vi "CMCryoControl.vi"() -> ()   [LabVIEW 2017]
uses:
  Globals/globals.vi
  Commands/ScanInterfaceGlobalData.vi
  Types/ScanInfo.ctl
panel:
  in  "Tab Control":enum32{"Control", "Measurements", "Defenitions"}(tab)
  in  "positionTrack":bool=TRUE
  in  "positionGO":bool
  in  "Position Info":cluster{"X":dbl, "Y":dbl} {"Y" step=0.01; "X" step=0.01}
  in  "StartStream":bool
  in  "Scan Info":T1={"X Center"=0.0, "Y Center"=0.0, "Width"=1.0, "Height"=1.0, "Time [ms]"=1000.0, "As Dwell Time"=FALSE, "Pixels"=1000.0}
  in  "ScanBtn":bool
  in  "Experiment List":i32(listbox)
  in  "Experiment Grps":u16(ring) items=["Sequential", "Time Resolved"]
  in  "StreamRate":dbl=10000.0
  in  "VI Search Path":path=path "C:/Code/CMCryoSysLabView/Experiments"
  out "CurrentReadAmplitude":dbl=50.013
  in  "Notifiers":T2
  out "Working":bool
  in  "IntensitySave":bool
  in  "IntensityLogScale":bool
  out "ScanImage":dbl[][](graph)
  in  "StreamSave":bool
  in  "StreamLogScale":bool
  out "Counter Trace":waveform(dbl)(graph)={"t0"=timestamp(1099.9 s since 1904-01-01), "dt"=0.09999999999990905, "Y"=array[30001 elements]}
  # "Dbl click to open experiment (or select and press open)"
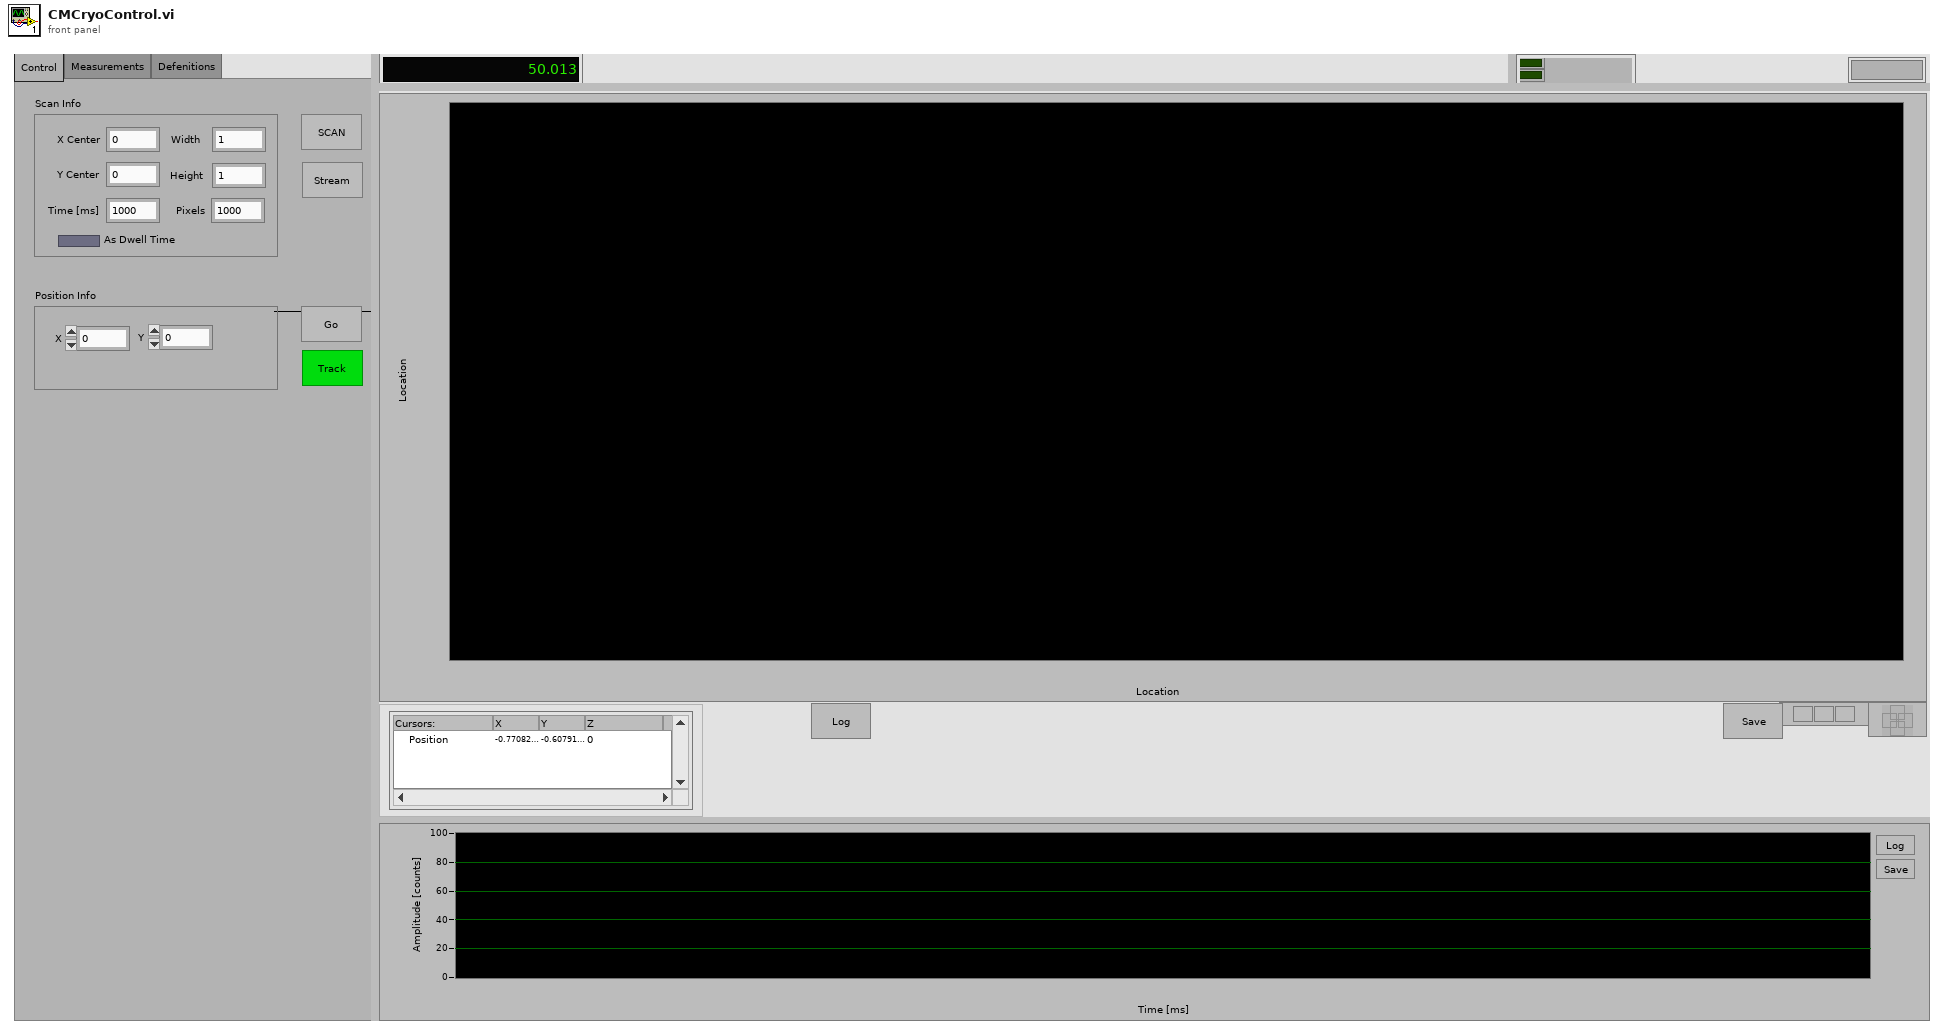
[diagram p1: front panel]
types:
  T1 = typedef "ScanInfo.ctl" = cluster{"X Center":dbl, "Y Center":dbl, "Width":dbl, "Height":dbl, "Time [ms]":dbl, "As Dwell Time":bool, "Pixels":dbl}
  T2 = cluster{"ImageCompleted":bool, "ImageUpdated":bool}
  T3 = typedef "ExperimentGrp.ctl" = cluster{"Path":path, "Experiments":path[], "Name":string, "Experiment Names":string[]}
  T4 = typedef "NotificationsInfo.ctl" = cluster{"ImageComplete":bool}
  T5 = typedef "StreamInfo.ctl" = cluster{"Waveform":waveform(dbl), "isNew":bool, "MeanV":dbl}
  T6 = typedef "ImageInfo.ctl" = cluster{"IsNew":bool, "Data":dbl[][], "XOffset":dbl, "YOffset":dbl, "dy":dbl, "dx":dbl, "xmin":dbl, "xmax":dbl, "ymin":dbl, "ymax":dbl, "width":dbl, "height":dbl, "whRatio":dbl}
  T7 = typedef "LVPoint32TypeDef.ctl" = cluster{"Horizontal":i32, "Vertical":i32}
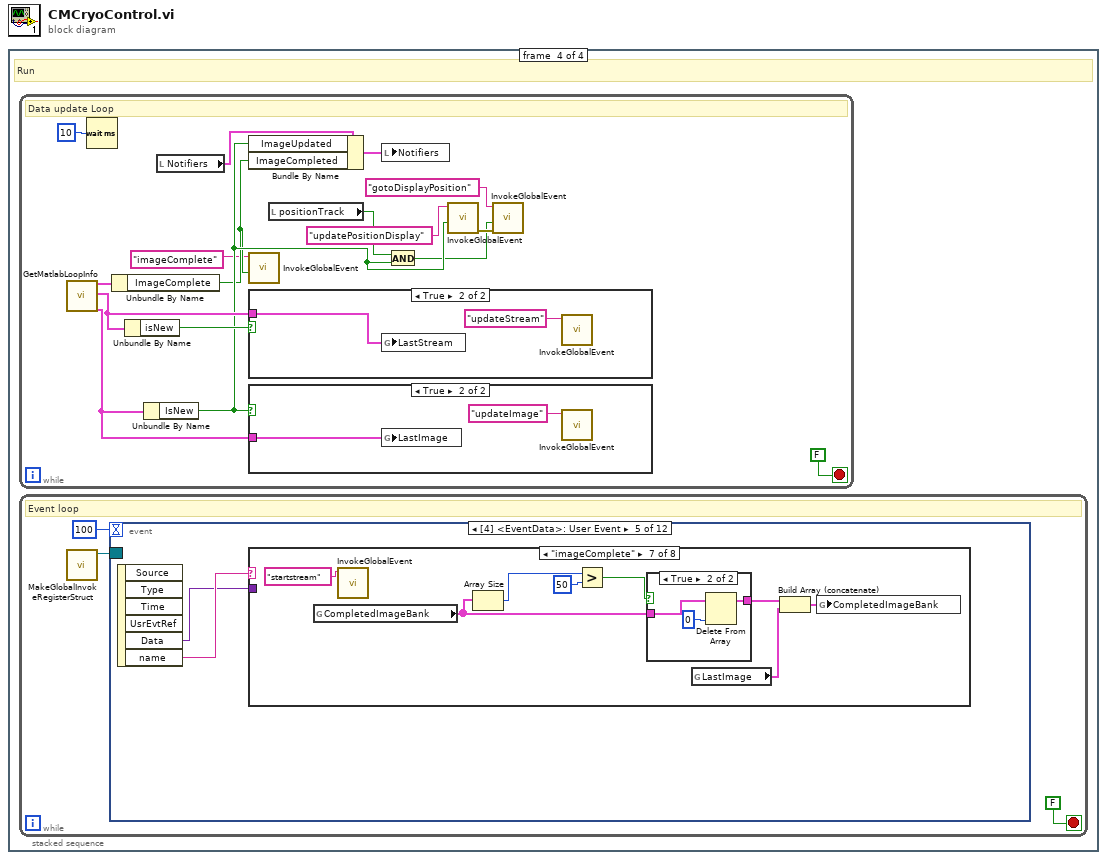
[diagram p0: block diagram]
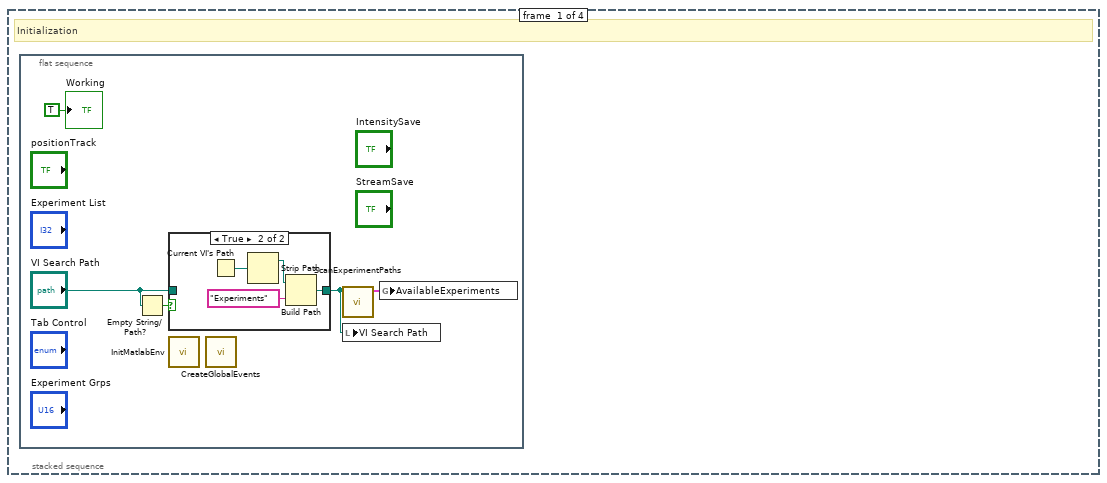
[diagram p2: hidden frame]
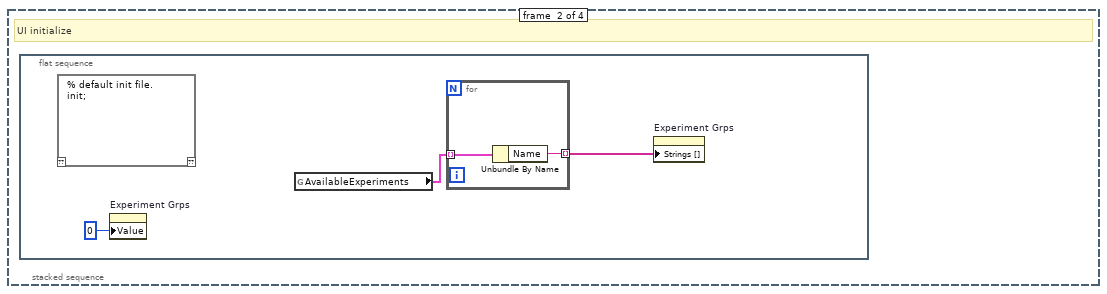
[diagram p4: hidden frame]
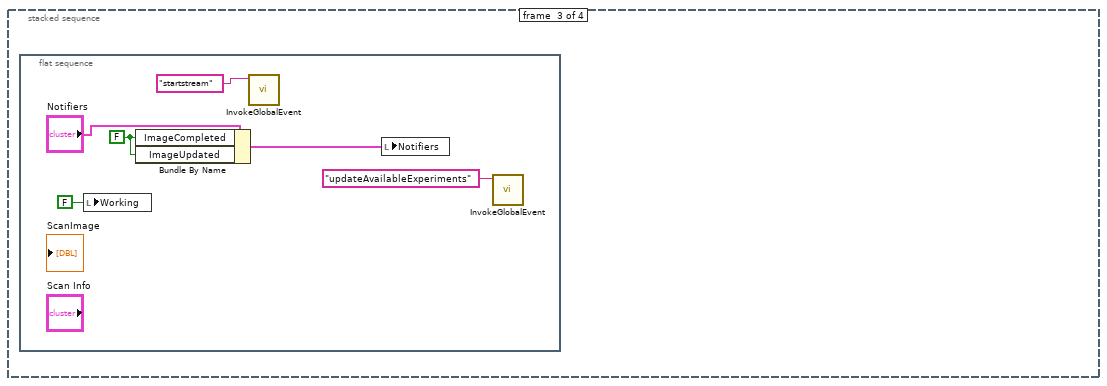
[diagram p5: hidden frame]
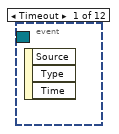
[diagram p8: hidden frame]
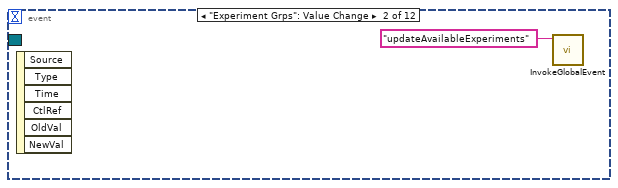
[diagram p9: hidden frame]
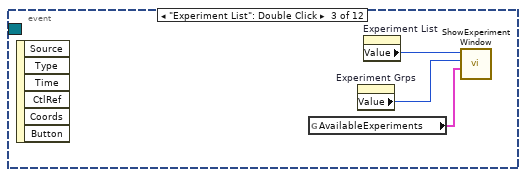
[diagram p10: hidden frame]
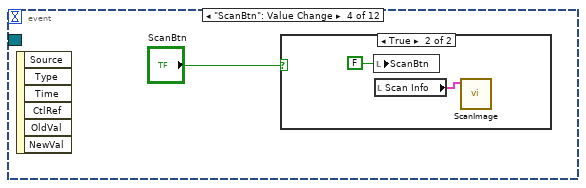
[diagram p11: hidden frame]
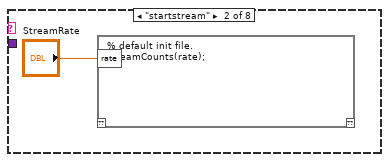
[diagram p14: hidden frame]
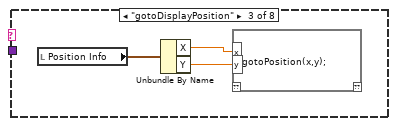
[diagram p15: hidden frame]
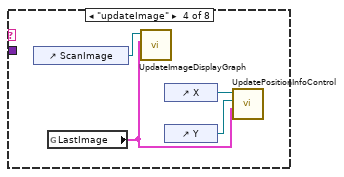
[diagram p16: hidden frame]
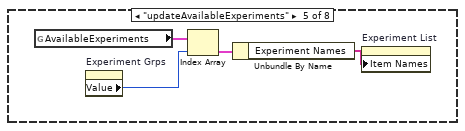
[diagram p17: hidden frame]
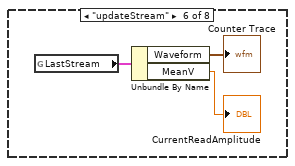
[diagram p18: hidden frame]
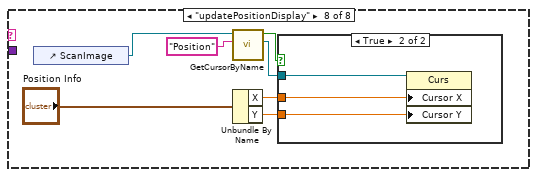
[diagram p20: hidden frame]
diagram:
  n1 = stacked-sequence {
    frame #0 {
      # "Initialization"
      n2 = flat-sequence {
        frame #0 {
          n3 = Empty String/Path?(string/path="VI Search Path") -> (empty?=w4:bool)
          n4 = case shown="True" w4 {
            tunnel: [w6 w8] -> w3
            tunnel: "VI Search Path" -> [w6 _]
            frame False {
            }
            frame True {
              n5 = Current VI's Path() -> (path=w7:path)
              n6 = Strip Path(path=w7) -> (stripped path=w10:path)  [unwired: 1 out]
              n7 = Build Path(base path=w10, name or relative path="Experiments") -> (appended path=w8:path)
            }
          }
          n8 = call "InitMatlabEnv.vi"() -> ()  [unwired: 12 in]
          n9 = call "CreateGlobalEvents.vi"() -> ()  [unwired: 12 in]
          n10 = call "ScanExperimentPaths.vi"("Scan path"=w3) -> ("AvailableExperiments"=w2:T3[])  [unwired: 10 in]
          n11 = local write "VI Search Path"(w3) -> ()
          n12 = global write "globals.vi" "AvailableExperiments"(w2) -> ()
          "Working" <- TRUE ("Status")
        }
      }
    }
    frame #1 {
      # "UI initialize"
      n13 = flat-sequence {
        frame #0 {
          n14 = script code="% default init file.\ninit;"() -> ()  [unwired: 1 in, 1 out]
          n15 = property on="Experiment Grps" class="Ring (strict)"("Value"=0 ("index")) -> ()  [unwired: 2 in, 2 out]
          n16 = global read "globals.vi" "AvailableExperiments"() -> (w13:T3[])
          n17 = for {
            tunnel: w13 -> [w15] mode=indexing
            tunnel: [w14] -> w12 mode=indexing
            n18 = Unbundle By Name(w15) -> ("Name"=w14:string)
          }
          n19 = property on="Experiment Grps" class="Ring (strict)"("Strings []"=w12) -> ()  [unwired: 2 in, 2 out]
        }
      }
    }
    frame #2 {
      n20 = flat-sequence {
        frame #0 {
          w19 = FALSE ("ImageCompleted")
          n21 = local write "Working"(FALSE ("Working")) -> ()
          n22 = Bundle By Name(cluster="Notifiers", "ImageCompleted"=w19, "ImageUpdated"=w19) -> (w20:T2)
          n23 = call "InvokeGlobalEvent.vi"("name"="startstream" ("event data")) -> ()  [unwired: 10 in, 1 out]
          n24 = local write "Notifiers"(w20) -> ()
          n25 = call "InvokeGlobalEvent.vi"("name"="updateAvailableExperiments" ("event data")) -> ()  [unwired: 10 in, 1 out]
        }
      }
    }
    frame #3 {
      # "Run"
      n26 = while {
        stop <- FALSE stop-if-true
        # "Data update Loop"
        n27 = call "GetMatlabLoopInfo.vi"() -> ("Notifications"=w33:T4, "StreamInfo"=w30:T5, "ImageInfo"=w29:T6)  [unwired: 17 in]
        n28 = Wait (ms)(milliseconds to wait=u32 10) -> ()  [unwired: 1 out]
        n29 = Unbundle By Name(w33) -> ("ImageComplete"=w23:bool)
        n30 = Unbundle By Name(w30) -> ("isNew"=w28:bool)
        n31 = Unbundle By Name(w29) -> ("IsNew"=w27:bool)
        n32 = local read "Notifiers"() -> (w35:T2)
        n33 = Bundle By Name(cluster=w35, "ImageUpdated"=w27, "ImageCompleted"=w23) -> (w34:T2)
        n34 = call "InvokeGlobalEvent.vi"("Invoke?"=w23, "name"="imageComplete" ("event data")) -> ()  [unwired: 9 in, 1 out]
        n35 = case shown="True" w28 {
          tunnel: w30 -> [_ w41]
          frame False {
          }
          frame True {
            n36 = global write "ScanInterfaceGlobalData.vi" "LastStream"(w41) -> ()
            n37 = call "InvokeGlobalEvent.vi"("name"="updateStream" ("event data")) -> ()  [unwired: 10 in, 1 out]
          }
        }
        n38 = case shown="True" w27 {
          tunnel: w29 -> [_ w39]
          frame False {
          }
          frame True {
            n39 = global write "ScanInterfaceGlobalData.vi" "LastImage"(w39) -> ()
            n40 = call "InvokeGlobalEvent.vi"("name"="updateImage" ("event data")) -> ()  [unwired: 10 in, 1 out]
          }
        }
        n41 = local read "positionTrack"() -> (w32:bool)
        n42 = local write "Notifiers"(w34) -> ()
        n43 = And(x=w32, y=w27) -> (x .and. y?=w26:bool)
        n44 = call "InvokeGlobalEvent.vi"("Invoke?"=w27, "name"="updatePositionDisplay" ("event data")) -> ("error out"=w31:errorcluster)  [unwired: 9 in]
        n45 = call "InvokeGlobalEvent.vi"("error in (no error)"=w31, "Invoke?"=w26, "name"="gotoDisplayPosition" ("event data")) -> ()  [unwired: 8 in, 1 out]
      }
      n46 = while {
        stop <- FALSE stop-if-true
        # "Event loop"
        n47 = call "MakeGlobalInvokeRegisterStruct.vi"() -> ("Event Registration Refnum out"=w42:refnum<event-registration>)  [unwired: 11 in]
        n48 = event shown="[4] <EventData>: User Event" {
          selector: w42 -> [_ _ _ _ _ _ _ _ _ _ _ _]
          dyn-events: _ -> [_ _ _ _ _ _ _ _ _ _ _ _]
          timeout: 100 -> [_ _ _ _ _ _ _ _ _ _ _ _]
          event Timeout {
            n49 = event-data() -> ()  [unwired: 1 in, 3 out]
          }
          event "Experiment Grps": Value Change {
            n50 = event-data() -> ()  [unwired: 1 in, 6 out]
            n51 = call "InvokeGlobalEvent.vi"("name"="updateAvailableExperiments" ("event data")) -> ()  [unwired: 10 in, 1 out]
          }
          event "Experiment List": Double Click {
            n52 = event-data() -> ()  [unwired: 1 in, 6 out]
            n53 = global read "globals.vi" "AvailableExperiments"() -> (w48:T3[])
            n54 = property on="Experiment Grps" class="Ring (strict)"() -> ("Value"=w46:u16)  [unwired: 2 in, 2 out]
            n55 = property on="Experiment List" class="LstBox (strict)"() -> ("Value"=w47:i32)  [unwired: 2 in, 2 out]
            n56 = call "ShowExperimentWindow.vi"("AvailableExperiments"=w48, "Value"=w46, "Value 2"=w47) -> ()  [unwired: 9 in]
          }
          event "ScanBtn": Value Change {
            n57 = event-data() -> ()  [unwired: 1 in, 6 out]
            n58 = case shown="True" "ScanBtn" {
              frame False {
              }
              frame True {
                n59 = local write "ScanBtn"(FALSE ("ScanBtn")) -> ()
                n60 = local read "Scan Info"() -> (w50:T1)
                n61 = call "ScanImage.vi"("Scan Info"=w50) -> ()  [unwired: 11 in]
              }
            }
          }
          event User Event {
            n62 = event-data() -> ("Data"=w52:variant, "name"=w53:string)  [unwired: 1 in, 4 out]
            n63 = case shown="\"imageComplete\"" w53 {
              tunnel: w52 -> [_ _ _ _ _ _ _ _]
              frame "False", Default {
              }
              frame "startstream" {
                n64 = script code="% default init file.\nstreamCounts(rate);"("rate"="StreamRate") -> ()  [unwired: 1 in, 1 out]
              }
              frame "gotoDisplayPosition" {
                n65 = local read "Position Info"() -> (w57:cluster{"X":dbl, "Y":dbl})
                n66 = Unbundle By Name(w57) -> ("X"=w56:dbl, "Y"=w55:dbl)
                n67 = script code="gotoPosition(x,y);"("x"=w56, "y"=w55) -> ()  [unwired: 1 in, 1 out]
              }
              frame "updateImage" {
                n68 = control-ref of="ScanImage"() -> (w59:refnum<vi>)
                n69 = global read "ScanInterfaceGlobalData.vi" "LastImage"() -> (w58:T6)
                n70 = call "UpdateImageDisplayGraph.vi"("ImageInfo"=w58, "IntensityGraph in"=w59) -> ()  [unwired: 10 in]
                n71 = control-ref of="X"() -> (w60:refnum<vi>)
                n72 = control-ref of="Y"() -> (w61:refnum<vi>)
                n73 = call "UpdatePositionInfoControl.vi"("ImageInfo"=w58, "Y"=w61, "Digital in"=w60) -> ()  [unwired: 9 in]
              }
              frame "updateAvailableExperiments" {
                n74 = global read "globals.vi" "AvailableExperiments"() -> (w63:T3[])
                n75 = property on="Experiment Grps" class="Ring (strict)"() -> ("Value"=w62:u16)  [unwired: 2 in, 2 out]
                n76 = Index Array(array=w63, index=w62) -> (element=w64:T3)
                n77 = Unbundle By Name(w64) -> ("Experiment Names"=w65:string[])
                n78 = property on="Experiment List" class="LstBox (strict)"("Item Names"=w65) -> ()  [unwired: 2 in, 2 out]
              }
              frame "updateStream" {
                n79 = global read "ScanInterfaceGlobalData.vi" "LastStream"() -> (w66:T5)
                n80 = Unbundle By Name(w66) -> ("Waveform"=→"Counter Trace":waveform(dbl), "MeanV"=→"CurrentReadAmplitude":dbl)
              }
              frame "imageComplete" {
                n81 = global read "ScanInterfaceGlobalData.vi" "CompletedImageBank"() -> (w71:T6[])
                n82 = call "InvokeGlobalEvent.vi"("name"="startstream" ("event data")) -> ()  [unwired: 10 in, 1 out]
                n83 = Array Size(array=w71) -> (size(s)=w74:i32)
                n84 = Greater?(x=w74, y=50) -> (0:w72:bool)
                n85 = case shown="True" w72 {
                  tunnel: w71 -> [w77 w80]
                  tunnel: [w77 w78] -> w70
                  frame False {
                  }
                  frame True {
                    n86 = Delete From Array(array=w80, index=0) -> (array with subset deleted=w78:T6[])  [unwired: 1 in, 1 out]
                  }
                }
                n87 = global read "ScanInterfaceGlobalData.vi" "LastImage"() -> (w76:T6)
                n88 = Build Array (concatenate)(w70, w76) -> (w75:T6[])
                n89 = global write "ScanInterfaceGlobalData.vi" "CompletedImageBank"(w75) -> ()
              }
              frame "updatePositionDisplay" {
                n90 = control-ref of="ScanImage"() -> (w87:refnum<vi>)
                n91 = call "GetCursorByName.vi"("Name"="Position", "IntensityGraph in"=w87) -> ("CursorRef"=w82:refnum<vi>, "Found?"=w81:bool)  [unwired: 7 in, 1 out]
                n92 = Unbundle By Name("Position Info") -> ("X"=w84:dbl, "Y"=w83:dbl)
                n93 = case shown="True" w81 {
                  tunnel: w84 -> [_ w90]
                  tunnel: w83 -> [_ w89]
                  tunnel: w82 -> [_ w88]
                  frame False {
                  }
                  frame True {
                    n94 = property class="Curs"(reference=w88, "Cursor X"=w90, "Cursor Y"=w89) -> ()  [unwired: 1 in, 2 out]
                  }
                }
              }
            }
          }
          event "Position Info": Value Change {
            n95 = event-data() -> ()  [unwired: 1 in, 6 out]
            n96 = local read "positionTrack"() -> (w92:bool)
            n97 = call "InvokeGlobalEvent.vi"("name"="updatePositionDisplay" ("event data")) -> ("error out"=w93:errorcluster)  [unwired: 10 in]
            n98 = case shown="True" w92 {
              tunnel: w93 -> [_ _]
              frame False {
              }
              frame True {
                n99 = call "InvokeGlobalEvent.vi"("name"="gotoDisplayPosition" ("event data")) -> ()  [unwired: 10 in, 1 out]
              }
            }
          }
          event "ScanImage": Mouse Up {
            n100 = event-data() -> ("Coords"=w103:T7)  [unwired: 1 in, 7 out]
            n101 = invoke on="ScanImage" class="IntGraph (strict)" method="Map Coords To XY"("Coords"=w103) -> ("XY"=w101:cluster{"X":dbl, "Y":dbl})  [unwired: 6 in, 6 out]
            n102 = local read "positionTrack"() -> (w96:bool)
            n103 = Unbundle By Name(w101) -> ("X"=w100:dbl, "Y"=w99:dbl)
            n104 = local read "Position Info"() -> (w102:cluster{"X":dbl, "Y":dbl})
            n105 = Bundle By Name(cluster=w102, "X"=w100, "Y"=w99) -> (w98:cluster{"X":dbl, "Y":dbl})
            n106 = call "InvokeGlobalEvent.vi"("name"="updatePositionDisplay" ("event data")) -> ()  [unwired: 10 in, 1 out]
            n107 = local write "Position Info"(w98) -> ()
            n108 = call "InvokeGlobalEvent.vi"("Invoke?"=w96, "name"="gotoDisplayPosition" ("event data")) -> ()  [unwired: 9 in, 1 out]
          }
          event "StreamLogScale": Value Change {
            n109 = event-data() -> ()  [unwired: 1 in, 6 out]
            n110 = call "InvokeGlobalEvent.vi"("name"="updateStream" ("event data")) -> ()  [unwired: 10 in, 1 out]
            n111 = Boolean To (0,1)(Boolean="StreamLogScale") -> (0, 1=w105:i16)
            n112 = property on="Counter Trace" class="WFGraph (strict)"("YScale.Mapping Mode"=w105) -> ()  [unwired: 2 in, 2 out]
          }
          event "IntensityLogScale": Value Change {
            n113 = event-data() -> ()  [unwired: 1 in, 6 out]
            n114 = call "InvokeGlobalEvent.vi"("name"="updateImage" ("event data")) -> ()  [unwired: 10 in, 1 out]
            n115 = Boolean To (0,1)(Boolean="IntensityLogScale") -> (0, 1=w108:i16)
            n116 = property on="ScanImage" class="IntGraph (strict)"("ZScale.Mapping Mode"=w108) -> ()  [unwired: 2 in, 2 out]
          }
          event "ScanImage": Cursor Move {
            n117 = event-data() -> ("CursRef"=w117:refnum<vi>)  [unwired: 1 in, 7 out]
            n118 = property class="Curs"(reference=w117) -> (reference out=w112:refnum<vi>, "Cursor Name"=w114:string)  [unwired: 1 in, 1 out]
            n119 = local read "positionTrack"() -> (w110:bool)
            n120 = local read "Position Info"() -> (w113:cluster{"X":dbl, "Y":dbl})
            n121 = Equal?(x=w114, y="Position") -> (x = y?=w115:bool)
            n122 = case shown="True" w115 {
              tunnel: w113 -> [_ w122]
              tunnel: w110 -> [_ _]
              tunnel: w112 -> [_ w120]
              frame False {
              }
              frame True {
                n123 = property class="Curs"(reference=w120) -> ("Cursor X"=w119:dbl, "Cursor Y"=w118:dbl)  [unwired: 1 in, 2 out]
                n124 = Bundle By Name(cluster=w122, "X"=w119, "Y"=w118) -> (w121:cluster{"X":dbl, "Y":dbl})
                n125 = local write "Position Info"(w121) -> ()
              }
            }
            n126 = call "InvokeGlobalEvent.vi"("Invoke?"=w110, "name"="gotoDisplayPosition" ("event data")) -> ()  [unwired: 9 in, 1 out]
          }
          event "positionGO": Value Change {
            n127 = event-data() -> ()  [unwired: 1 in, 6 out]
            n128 = case shown="True" "positionGO" {
              frame False {
              }
              frame True {
                n129 = local write "positionGO"(FALSE ("positionGO")) -> ()
                n130 = call "InvokeGlobalEvent.vi"("name"="gotoDisplayPosition" ("event data")) -> ()  [unwired: 10 in, 1 out]
              }
            }
          }
          event "StartStream": Value Change {
            n131 = event-data() -> ()  [unwired: 1 in, 6 out]
            n132 = case shown="True" "StartStream" {
              frame False {
              }
              frame True {
                n133 = local write "StartStream"(FALSE ("StartStream")) -> ()
                n134 = call "InvokeGlobalEvent.vi"("name"="startstream" ("event data")) -> ()  [unwired: 10 in, 1 out]
              }
            }
          }
        }
      }
    }
  }
